vi "Лабораторная №1 Задание 3_10.vi"() -> ()   [LabVIEW 2017]
panel:
  out "Square root":string
  in  "Dial":dbl(knob) scale=-10.0..10.0
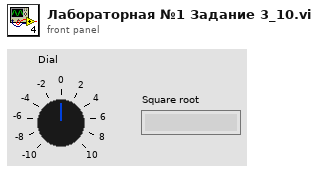
[diagram p1: front panel]
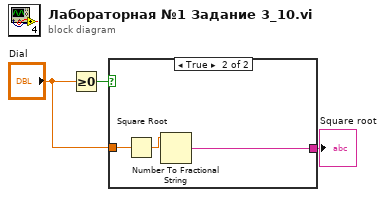
[diagram p0: block diagram]
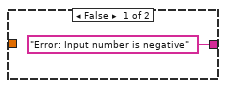
[diagram p2: hidden frame]
diagram:
  n1 = Greater Or Equal To 0?(x="Dial") -> (x >= 0?=w3:bool)
  n2 = case shown="True" w3 {
    tunnel: "Dial" -> [_ w7]
    tunnel: ["Error: Input number is negative" w6] -> w1
    frame False {
    }
    frame True {
      n3 = Square Root(x=w7) -> (sqrt(x)=w5:dbl)
      n4 = Number To Fractional String(number=w5) -> (F-format string=w6:string)  [unwired: 3 in]
    }
  }
  "Square root" <- w1
